vi "New649DigitGen.vi"(2 "const + StdAvr":dbl) -> (0 "2D ResUArr - STD of each row is equal to (Last STD - Avr STD)":u64[][](array[numeric]), 1 "Waveform Graph":dbl[][](graph), 3 "CurrAvrSTDToArr - only six":dbl[](array[numeric]) format="%#_4f", 4 "lastStd":dbl format="%#_4g")   [LabVIEW 2023]
panel:
  out "1D Std":dbl[](array[numeric])
  out "size(s)":i32
  out "Size(s)":i32
  out "Last STD":dbl format="%#_3g"
  out "Avr STD":dbl
  out "Std":dbl[](array[numeric]) format="%#_4g"
  out "AvrSTDtoArray - All":dbl[](array[numeric]) format="%#_4g"
  out "LastSTDToArray":dbl[](array[numeric])
  out "Row Std":dbl[](array[numeric]) format="%#_3f"
  out "Java file - official result":i64[][](array[numeric])
  # "Генерира масив всеки ред на който е с STD = AvrResultsSTD +/- N"
  # "K"
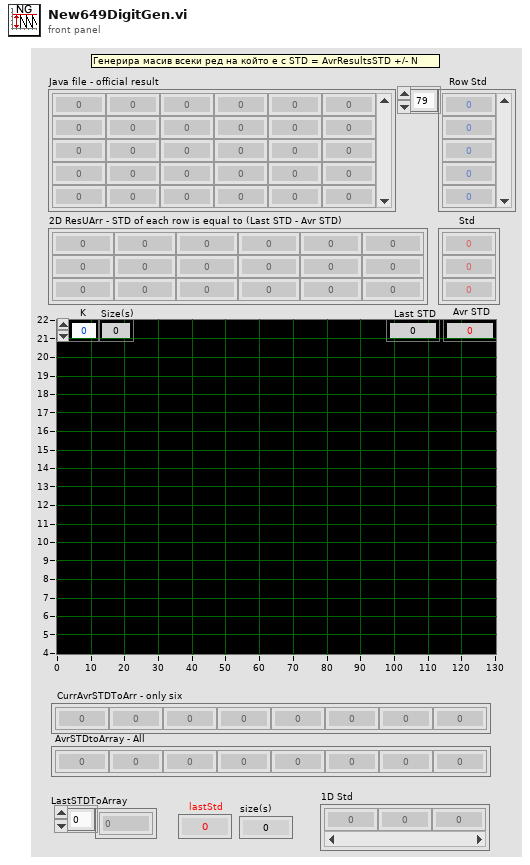
[diagram p1: front panel]
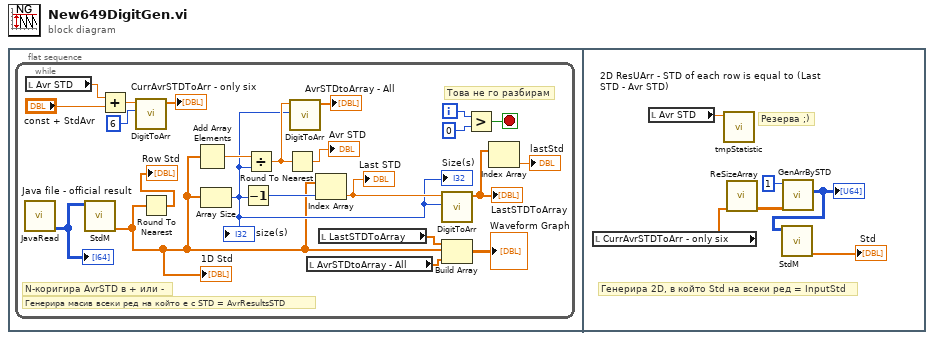
[diagram p0: block diagram]
diagram:
  n1 = flat-sequence {
    frame #0 {
      n2 = while {
        i -> [w15]
        stop <- w13 stop-if-true
        # "Това не го разбирам"
        # "N-коригира AvrSTD в + или -"
        # "Генерира масив всеки ред на който е с STD = AvrResultsSTD"
        n3 = call "JavaRead.vi"() -> ("Java file"=w23:i64[][])  [unwired: 10 in, 1 out]
        "Java file - official result" <- w23
        n4 = local read "Avr STD"() -> (w9:dbl)
        n5 = call "StdM.vi"("2D in"=w23) -> ("1D Std"=w1:dbl[])  [unwired: 6 in, 4 out]
        "1D Std" <- w1
        n6 = Add(x=w9, y="const + StdAvr") -> (x+y=w6:dbl)
        n7 = call "DigitToArr.vi"("Arr Size"=6, "Digit"=w6) -> ("Array out"=→"CurrAvrSTDToArr - only six":dbl[])  [unwired: 9 in]
        n8 = Round To Nearest(number=w1) -> (nearest integer value=→"Row Std":dbl[])
        n9 = Add Array Elements(numeric array=w1) -> (sum=w22:dbl)
        n10 = Array Size(array=w1) -> (size(s)=w7:i32)
        "Size(s)" <- w7
        "size(s)" <- w7
        n11 = Decrement(x=w7) -> (x-1=w2:i32)
        n12 = Divide(x=w22, y=w7) -> (x/y=w12:dbl)
        n13 = Round To Nearest(number=w12) -> (nearest integer value=→"Avr STD":dbl)
        n14 = call "DigitToArr.vi"("Arr Size"=w7, "Digit"=w12) -> ("Array out"=→"AvrSTDtoArray - All":dbl[])  [unwired: 9 in]
        n15 = local read "AvrSTDtoArray - All"() -> (w5:dbl[])
        n16 = Index Array(array=w1, index=w2) -> (element=w20:dbl)
        "Last STD" <- w20
        n17 = local read "LastSTDToArray"() -> (w18:dbl[])
        n18 = call "DigitToArr.vi"("Arr Size"=w7, "Digit"=w20) -> ("Array out"=w4:dbl[])  [unwired: 9 in]
        "LastSTDToArray" <- w4
        n19 = Build Array(w18, w1, w5) -> (→"Waveform Graph":dbl[][])
        n20 = Greater?(x=w15, y=0) -> (0:w13:bool)
        n21 = Index Array(array=w4) -> (element=→"lastStd":dbl)  [unwired: 1 in]
      }
    }
    frame #1 {
      # "Генерира 2D, в който Std на всеки ред = InputStd"
      # "Резерва ;)"
      n22 = local read "CurrAvrSTDToArr - only six"() -> (w25:dbl[])
      n23 = local read "Avr STD"() -> (w29:dbl)
      n24 = call "tmpStatistic.vi"("My Std"=w29) -> ()  [unwired: 10 in, 1 out]
      n25 = call "ReSizeArray.vi"("1D"=w25) -> ("2D"=w28:dbl[][])  [unwired: 9 in, 1 out]
      n26 = call "GenArrBySTD.vi"("2D Array"=w28, "Last idx -"=1) -> ("2D ResUArr"=w26:u64[][])  [unwired: 6 in, 3 out]
      "2D ResUArr - STD of each row is equal to (Last STD - Avr STD)" <- w26
      n27 = call "StdM.vi"("2D in"=w26) -> ("1D Std"=→"Std":dbl[])  [unwired: 6 in, 4 out]
    }
  }
